vi "Single Item Save Dark Current.vi"(8 "Filename":string, 9 "Voltage":dbl, 10 "Barcode":string, 11 "Current":dbl) -> ()   [LabVIEW 2020]
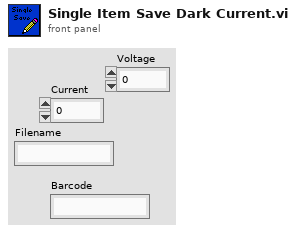
[diagram p1: front panel]
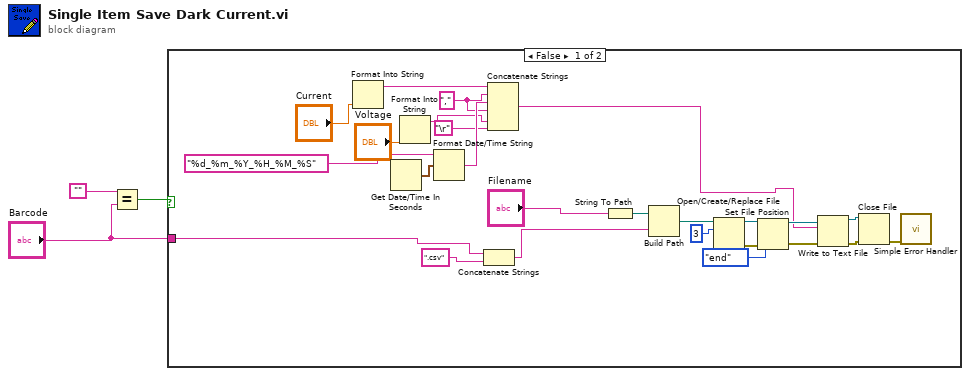
[diagram p0: block diagram]
diagram:
  n1 = Equal?(x="", y="Barcode") -> (x = y?=w3:bool)
  n2 = case shown="False" w3 {
    tunnel: "Barcode" -> [w19 _]
    frame False {
      w6 = ","
      n3 = Format Into String("Current") -> (resulting string=w27:string)  [unwired: 3 in, 1 out]
      n4 = Get Date/Time In Seconds() -> (seconds since 1Jan1904=w20:timestamp)
      n5 = Format Into String("Voltage") -> (resulting string=w4:string)  [unwired: 3 in, 1 out]
      n6 = Format Date/Time String(time format string (%c)="%d_%m_%Y_%H_%M_%S", seconds (now)=w20) -> (date/time string=w15:string)  [unwired: 1 in]
      n7 = Concatenate Strings(w19, ".csv" ("string")) -> (w16:string)
      n8 = Concatenate Strings(w27, w6, w15, w6, w4, "\r") -> (w9:string)
      n9 = String To Path(string="Filename") -> (path=w21:path)
      n10 = Build Path(base path=w21, name or relative path=w16) -> (appended path=w22:path)
      n11 = Open/Create/Replace File(file path (use dialog)=w22, operation (0:open)=3) -> (refnum out=w14:refnum<file>, error out=w13:errorcluster)  [unwired: 4 in, 1 out]
      n12 = Set File Position(refnum=w14, from (0:start)=enum16{"start", "end", "current"}."end", error in=w13) -> (refnum out=w11:refnum<file>, error out=w10:errorcluster)  [unwired: 1 in]
      n13 = Write to Text File(file (use dialog)=w11, text=w9, error in=w10) -> (refnum out=w23:refnum<file>, error out=w24:errorcluster)  [unwired: 1 in, 1 out]
      n14 = Close File(refnum=w23, error in=w24) -> (error out=w25:errorcluster)  [unwired: 1 out]
      n15 = call <vilib>:"Simple Error Handler.vi"("error in (no error)"=w25) -> ()  [unwired: 4 in, 5 out]
    }
    frame True {
    }
  }
